vi "Read Transmission Data Unit.vi"(8 "error in (no error)":errorcluster, 11 "Network Protocol in":refnum<class "Network Protocol.lvclass">) -> (0 "error out":errorcluster, 2 "Transmission Data Unit":refnum<class "Transmission Data Unit.lvclass">, 3 "Network Protocol out":refnum<class "Network Protocol.lvclass">)   [LabVIEW 2021, in "Network Protocol.lvclass"]
uses:
  Network Protocol.lvclass
  Network Protocol.lvclass/Network Protocol.ctl
  Transmission Data Unit/Transmission Data Unit.lvclass
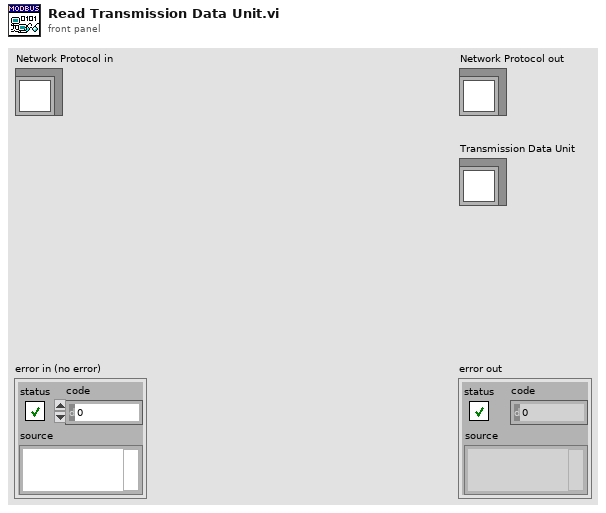
[diagram p1: front panel]
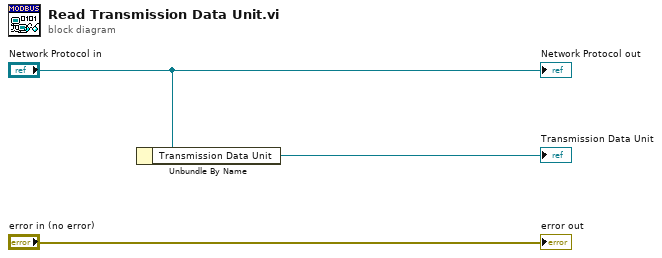
[diagram p0: block diagram]
diagram:
  n1 = Unbundle By Name("Network Protocol in") -> ("Transmission Data Unit"=→"Transmission Data Unit":refnum<class "Transmission Data Unit.lvclass">)
  "error out" <- "error in (no error)"
  "Network Protocol out" <- "Network Protocol in"
